vi "Hotel Room Service System.vi"() -> ()   [LabVIEW 2022 SP3]
uses:
  <vilib>/addons/control/pid/pid.llb/PID (DBL).vi
  <vilib>/addons/control/pid/NI_PID_pid.lvlib
panel:
  out "Emergency R2":bool
  in  "Smoke sensor":dbl(knob) scale=1.0..100.0 scale format="%#.6g"
  in  "Smoke sensor":dbl(knob) min=0.0 max=100.0 step=1.0 scale=0.0..100.0 scale format="%#.2g"
  in  "?":T1
  out "Password 3":string
  out "String 3":string
  out "Slide 2":u8(slide) scale=0.0..100.0
  in  "Search Button 2":bool
  out "Emergency R1":bool
  in  "Password 2":T1
  out "Password":string
  out "String 2":string
  out "Slide":u8(slide) scale=0.0..100.0
  in  "Search Button":bool
  in  "?":bool
  in  "Set point":dbl(slide)=15.0 min=15.0 max=30.0 step=1.0 scale=15.0..30.0
  in  "Room Tempreature":dbl(slide) scale=0.0..40.0
  out "System Action":string
  out "AC 3":bool
  out "Heator 6":bool
  in  "Set point":dbl(slide)=15.0 min=15.0 max=30.0 step=1.0 scale=15.0..30.0
  out "Heator":bool
  out "AC":bool
  out "System Action":string
  in  "A":dbl(slide) caption="Room Tempreature" min=0.0 max=45.0 step=1.0 scale=0.0..50.0
  in  "?":bool
  out "Your Order will be Prepared in":dbl
  out "R2":bool
  in  "Pay Bill and Conform":bool
  in  "Cheesecake":bool
  in  "Quantity":dbl=1.0 min=1.0 max=10.0 step=1.0
  out "Price":dbl
  in  "Chocolate Cake":bool
  in  "Quantity":dbl=1.0 min=1.0 max=10.0 step=1.0
  out "Price":dbl
  out "Total Bill":dbl
  out "Discount":string
  out "Order":string
  out "Order":string
  out "R1":bool
  out "Your Order will be Prepared in":dbl
  in  "Pay Bill and Conform":bool
  out "Discount":string
  out "Total Bill":dbl
  out "Price":dbl
  in  "Quantity 4":dbl=1.0 min=1.0 max=10.0 step=1.0
  in  "Chocolate Cake":bool
  out "Price":dbl
  in  "Quantity 3":dbl=1.0 min=1.0 max=10.0 step=1.0
  in  "Cheesecake":bool
  # "Hotel Room Service System"
  # "Customer Display"
  # "Hotel Display"
  # "Room 1"
  # "Foods"
  # "Room Tempreature Control"
  # "Room 2"
  # "Door Lock control"
  # "Door Lock control"
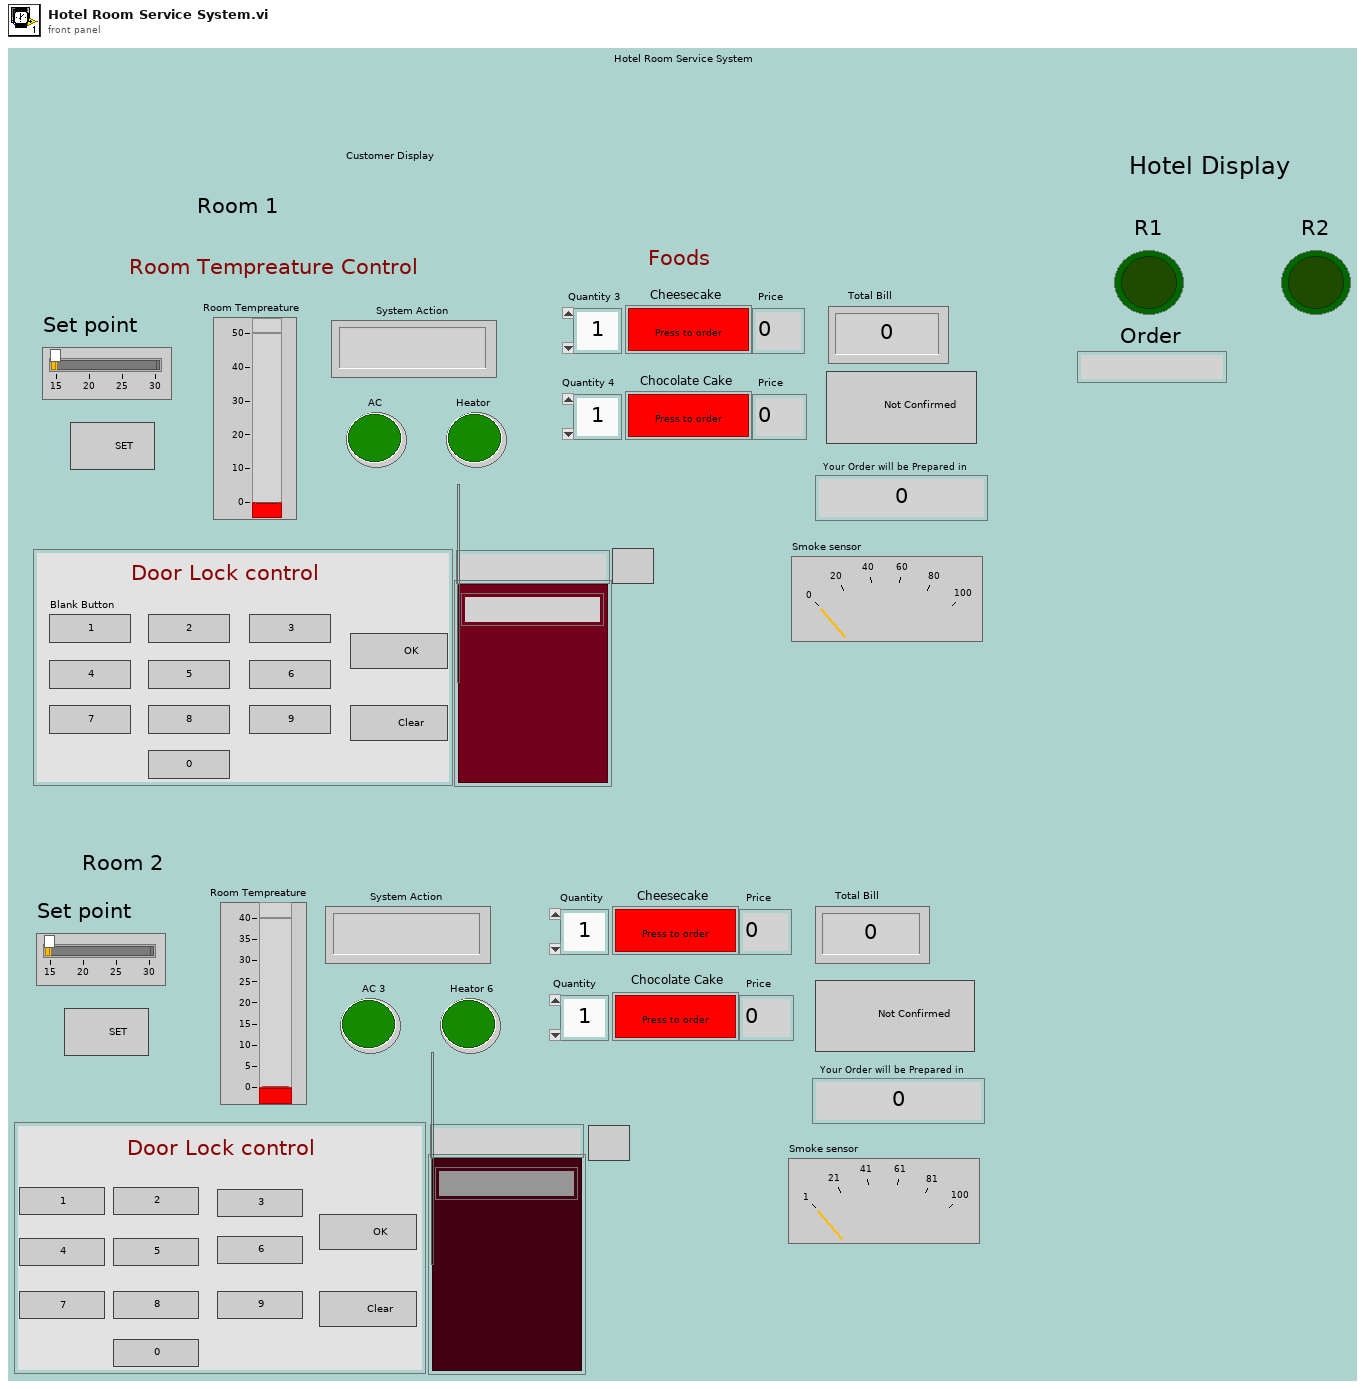
[diagram p1: front panel]
types:
  T1 = cluster{"Blank Button":bool, "Blank Button 2":bool, "Blank Button 3":bool, "Blank Button 4":bool, "Blank Button 5":bool, "Blank Button 6":bool, "Blank Button 7":bool, "Blank Button 8":bool, "Blank Button 9":bool, "Blank Button 10":bool, "OK Button":bool, "Refresh Button":bool}
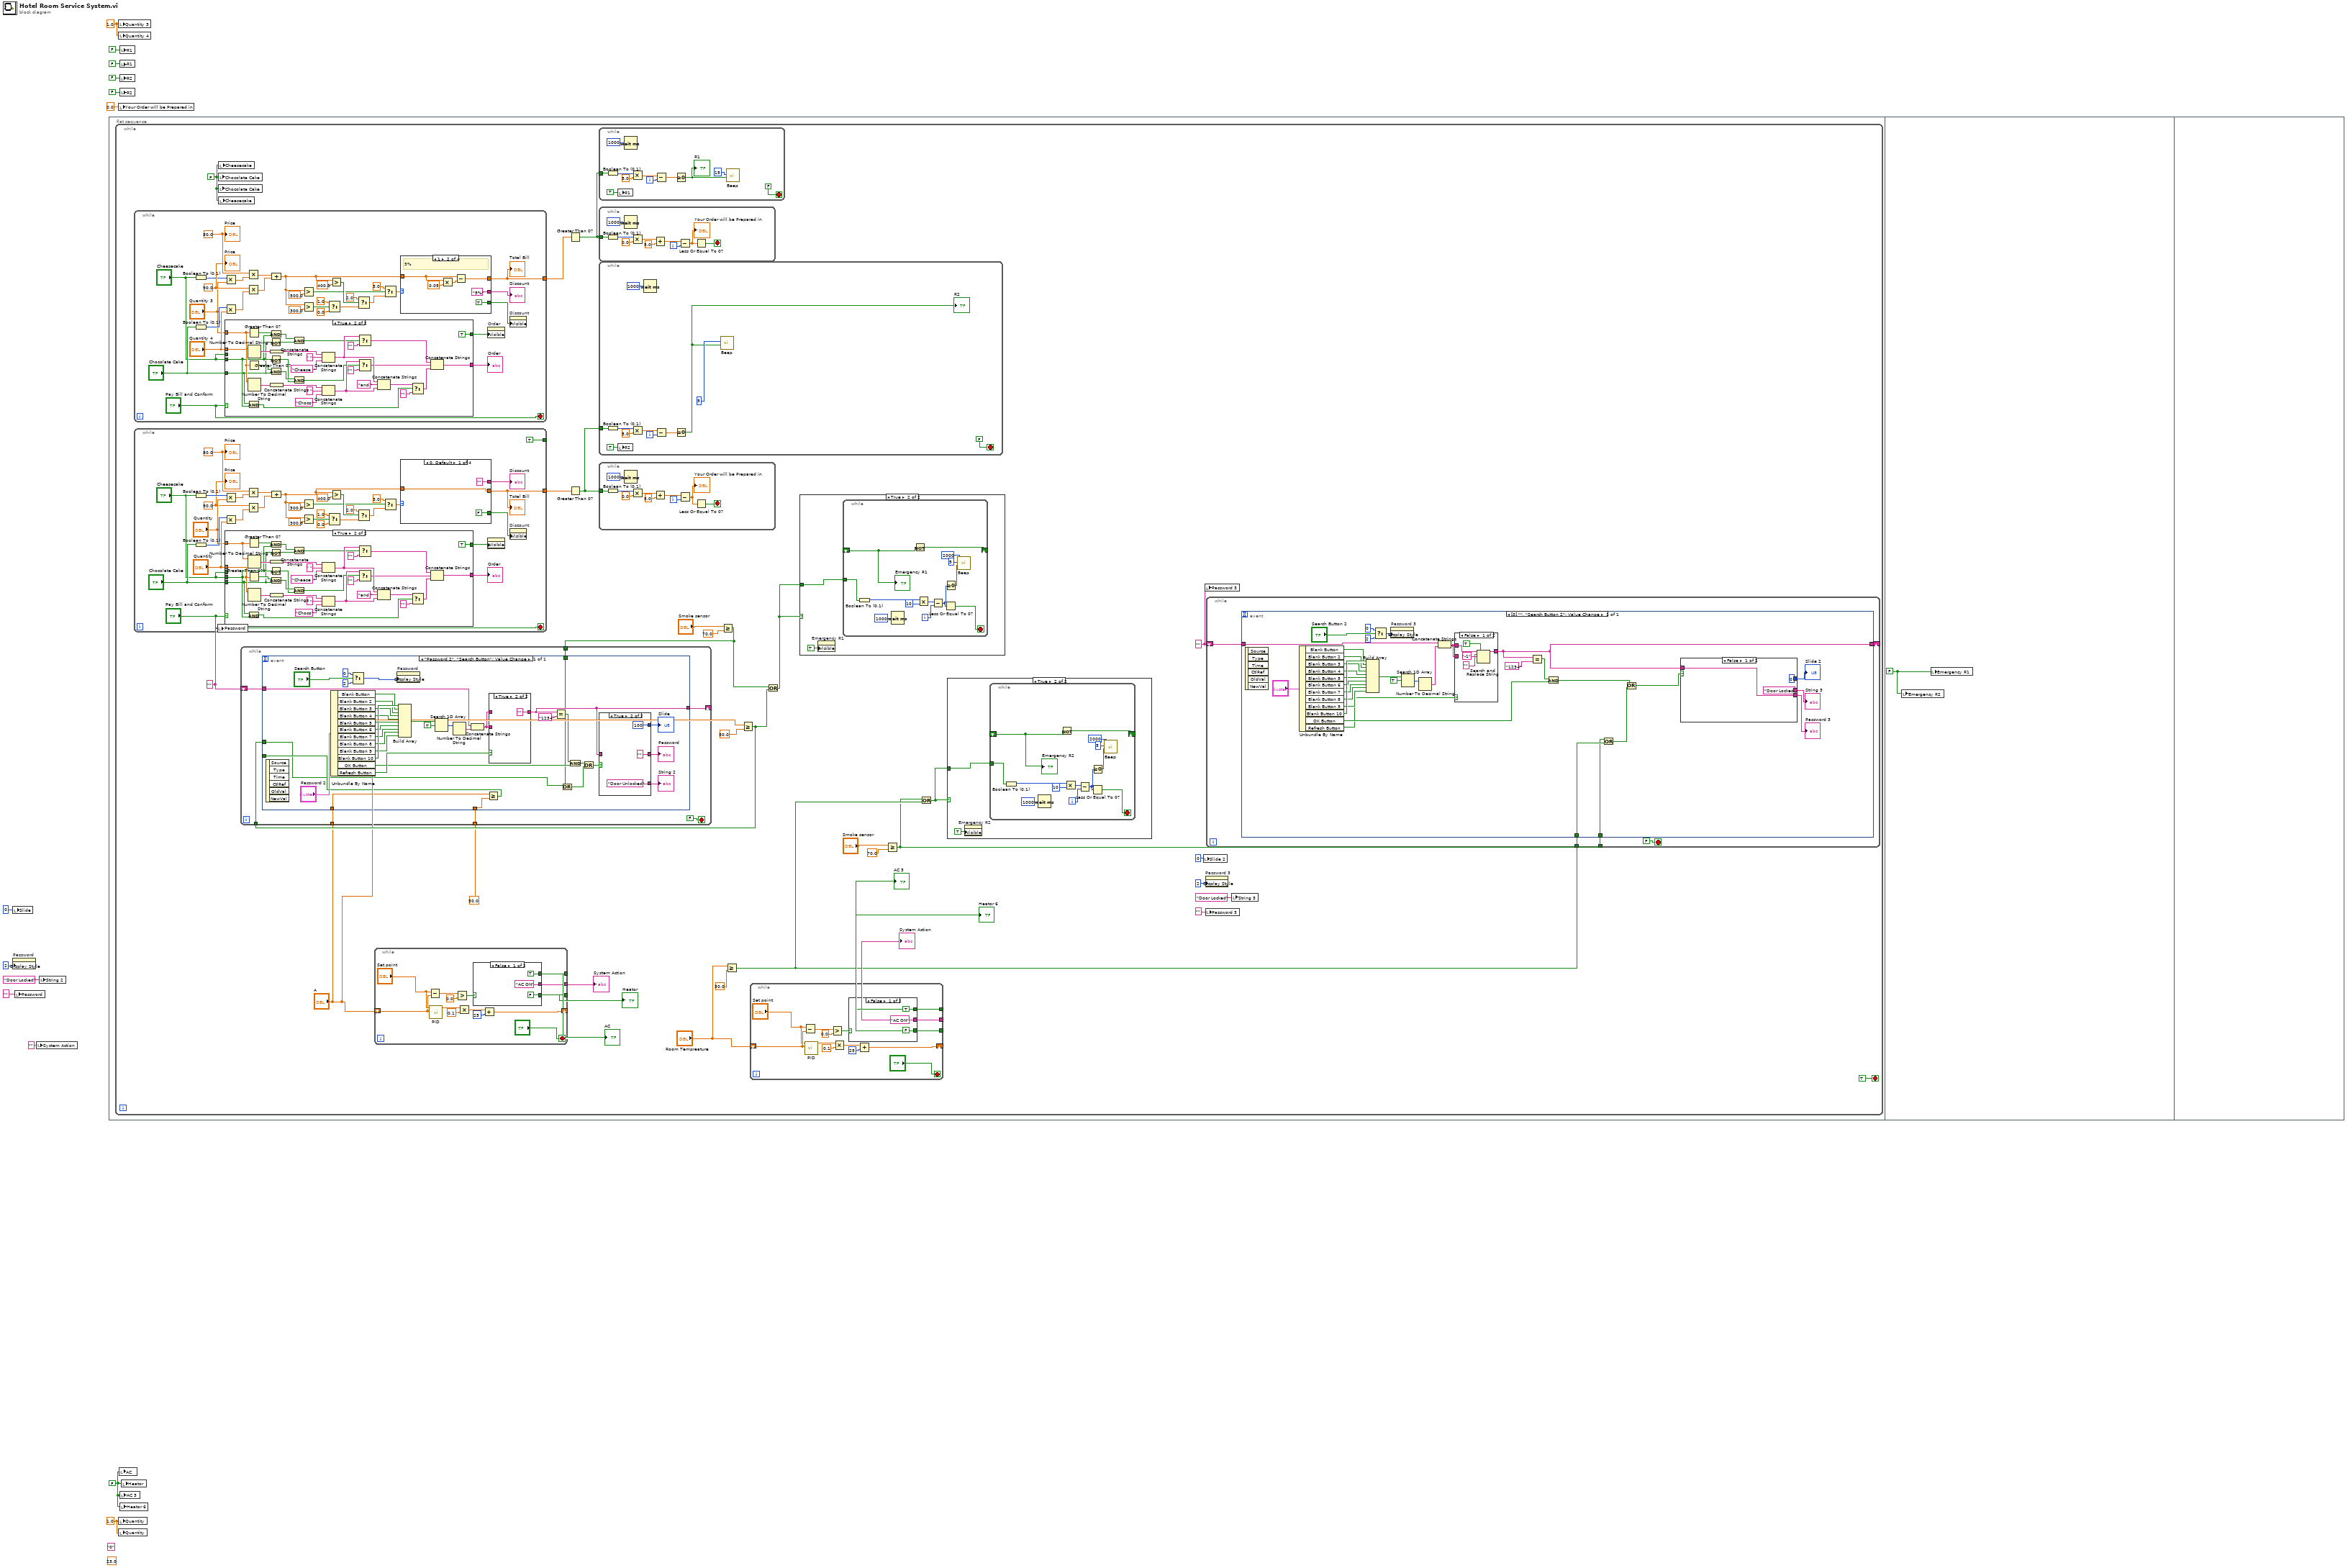
[diagram p0: block diagram]
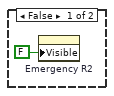
[diagram p2: hidden frame]
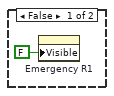
[diagram p3: hidden frame]
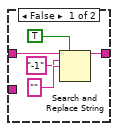
[diagram p4: hidden frame]
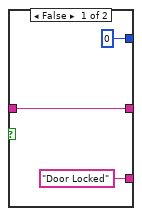
[diagram p5: hidden frame]
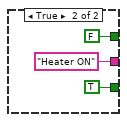
[diagram p6: hidden frame]
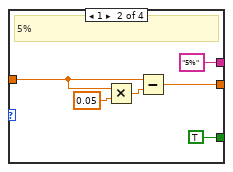
[diagram p7: hidden frame]
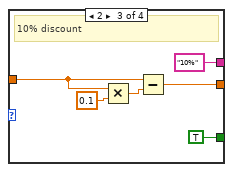
[diagram p8: hidden frame]
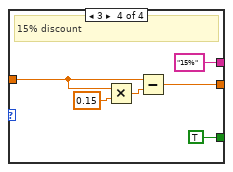
[diagram p9: hidden frame]
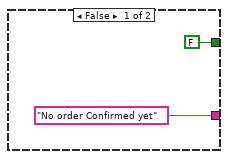
[diagram p10: hidden frame]
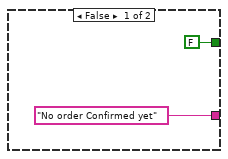
[diagram p11: hidden frame]
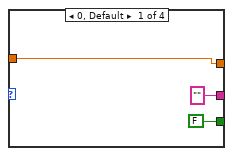
[diagram p12: hidden frame]
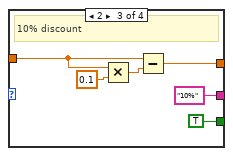
[diagram p13: hidden frame]
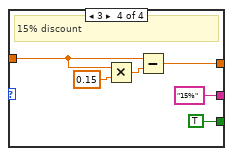
[diagram p14: hidden frame]
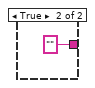
[diagram p15: hidden frame]
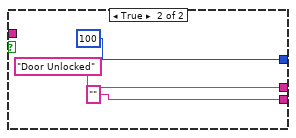
[diagram p16: hidden frame]
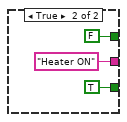
[diagram p17: hidden frame]
diagram:
  w6 = FALSE
  (unwired) 23.0 ("Target Temprature")
  (unwired) "0" ("Final")
  w9 = 1.0 ("Your Order will be Prepared in")
  w12 = 1.0 ("Your Order will be Prepared in")
  n1 = local write "Slide"(u8 0 ("Slide")) -> ()
  n2 = property on="Password" class="Str"("Display Style"=u32 2) -> ()  [unwired: 2 in, 2 out]
  n3 = local write "Password"("" ("Password")) -> ()
  n4 = local write "System Action"("" ("System Action")) -> ()
  n5 = local write "String 2"("Door Locked" ("String 2")) -> ()
  n6 = flat-sequence {
    frame #0 {
      n7 = while {
        stop <- TRUE stop-if-true
        w32 = ""
        w35 = ""
        w45 = FALSE ("Item 1")
        n8 = while {
          tunnel: [w295] -> w46
          stop <- "Pay Bill and Conform" stop-if-true
          w314 = 90.0 ("Price")
          w317 = 80.0 ("Price")
          n9 = Boolean To (0,1)(Boolean="Cheesecake") -> (0, 1=w294:i16)
          n10 = Boolean To (0,1)(Boolean="Chocolate Cake") -> (0, 1=w316:i16)
          n11 = Multiply(x=w294, y="Quantity 3") -> (x*y=w292:dbl)
          n12 = Multiply(x=w316, y="Quantity 4") -> (x*y=w315:dbl)
          n13 = case shown="True" "Pay Bill and Conform" {
            tunnel: ["No order Confirmed yet" w351] -> w293
            tunnel: "Quantity 4" -> [_ w347]
            tunnel: [FALSE TRUE ("Visible")] -> w291
            tunnel: "Quantity 3" -> [_ w329]
            tunnel: "Cheesecake" -> [_ _]
            tunnel: "Chocolate Cake" -> [_ w320]
            tunnel: "Cheesecake" -> [_ w321]
            frame False {
            }
            frame True {
              n14 = Greater Than 0?(x=w329) -> (x > 0?=w339:bool)
              n15 = Greater Than 0?(x=w347) -> (x > 0?=w338:bool)
              n16 = And(x=w320, y=w321) -> (x .and. y?=w337:bool)
              n17 = Number To Decimal String(number=w329) -> (decimal integer string=w350:string)  [unwired: 1 in]
              n18 = Number To Decimal String(number=w347) -> (decimal integer string=w349:string)  [unwired: 1 in]
              n19 = And(x=w339, y=w321) -> (x .and. y?=w325:bool)
              n20 = Not(x=w320) -> (.not. x?=w324:bool)
              n21 = Not(x=w321) -> (.not. x?=w328:bool)
              n22 = And(x=w338, y=w320) -> (x .and. y?=w330:bool)
              n23 = Concatenate Strings(w350) -> (w344:string)
              n24 = Concatenate Strings(w349) -> (w346:string)
              n25 = And(x=w325, y=w324) -> (x .and. y?=w323:bool)
              n26 = And(x=w330, y=w328) -> (x .and. y?=w322:bool)
              n27 = Concatenate Strings(w344, " ", "Cheese  ") -> (w335:string)
              n28 = Concatenate Strings(w346, " ", "Choco") -> (w333:string)
              n29 = Select(t=w335, s=w323, f="") -> (s? t:f=w327:string)
              n30 = Select(t=w333, s=w322, f="") -> (s? t:f=w326:string)
              n31 = Concatenate Strings(w335, "and ", w333) -> (w332:string)
              n32 = Select(t=w332, s=w337, f="") -> (s? t:f=w331:string)
              n33 = Concatenate Strings(w327, w326, w331) -> (w351:string)
            }
          }
          "Order" <- w293
          n34 = Multiply(x=w317, y=w292) -> (x*y=w313:dbl)
          n35 = Multiply(x=w314, y=w315) -> (x*y=w312:dbl)
          n36 = Compound Arithmetic op=ADD(w313, w312) -> (w298:dbl)
          n37 = Greater?(x=w298, y=500.0) -> (0:w300:bool)
          n38 = Greater?(x=w298, y=300.0) -> (0:w308:bool)
          n39 = Select(t=1.0, s=w308, f=0.0) -> (s? t:f=w303:dbl)
          n40 = Greater?(x=w298, y=400.0) -> (0:w305:bool)
          n41 = Select(t=2.0, s=w305, f=w303) -> (s? t:f=w301:dbl)
          n42 = Select(t=3.0, s=w300, f=w301) -> (s? t:f=w299:dbl)
          n43 = case shown="1" w299 {
            tunnel: w298 -> [w353 w359 w365 w371]
            tunnel: ["" ("Discount") "5%" ("Discount") "10%" ("Discount") "15%" ("Discount")] -> w297
            tunnel: [FALSE ("Visible") TRUE ("Visible") TRUE ("Visible") TRUE ("Visible")] -> w296
            tunnel: [w353 w356 w362 w368] -> w295
            frame 0, Default {
            }
            frame 1 {
              # "5%"
              n44 = Multiply(x=w359, y=0.05) -> (x*y=w360:dbl)
              n45 = Subtract(x=w359, y=w360) -> (x-y=w356:dbl)
            }
            frame 2 {
              # "10% discount"
              n46 = Multiply(x=w365, y=0.1) -> (x*y=w367:dbl)
              n47 = Subtract(x=w365, y=w367) -> (x-y=w362:dbl)
            }
            frame 3 {
              # "15% discount"
              n48 = Multiply(x=w371, y=0.15) -> (x*y=w373:dbl)
              n49 = Subtract(x=w371, y=w373) -> (x-y=w368:dbl)
            }
          }
          "Total Bill" <- w295
          "Discount" <- w297
          n50 = property on="Order" class="Str"("Visible"=w291) -> ()  [unwired: 2 in, 2 out]
          n51 = property on="Discount" class="Str"("Visible"=w296) -> ()  [unwired: 2 in, 2 out]
          "Price" <- w317
          "Price" <- w314
        }
        n52 = while {
          tunnel: [TRUE ("x")] -> _
          tunnel: [w197] -> w42
          stop <- "Pay Bill and Conform" stop-if-true
          w201 = 90.0 ("Price")
          w200 = 80.0 ("Price")
          n53 = Boolean To (0,1)(Boolean="Cheesecake") -> (0, 1=w216:i16)
          n54 = Boolean To (0,1)(Boolean="Chocolate Cake") -> (0, 1=w225:i16)
          n55 = Multiply(x=w216, y="Quantity") -> (x*y=w214:dbl)
          n56 = Multiply(x=w225, y="Quantity") -> (x*y=w224:dbl)
          n57 = case shown="True" "Pay Bill and Conform" {
            tunnel: ["No order Confirmed yet" w284] -> w215
            tunnel: "Quantity" -> [_ w280]
            tunnel: [FALSE TRUE ("Visible")] -> w213
            tunnel: "Quantity" -> [_ w262]
            tunnel: "Cheesecake" -> [_ _]
            tunnel: "Chocolate Cake" -> [_ w253]
            tunnel: "Cheesecake" -> [_ w254]
            frame False {
            }
            frame True {
              n58 = Greater Than 0?(x=w262) -> (x > 0?=w272:bool)
              n59 = Greater Than 0?(x=w280) -> (x > 0?=w271:bool)
              n60 = And(x=w253, y=w254) -> (x .and. y?=w270:bool)
              n61 = Number To Decimal String(number=w262) -> (decimal integer string=w283:string)  [unwired: 1 in]
              n62 = Number To Decimal String(number=w280) -> (decimal integer string=w282:string)  [unwired: 1 in]
              n63 = And(x=w272, y=w254) -> (x .and. y?=w258:bool)
              n64 = Not(x=w253) -> (.not. x?=w257:bool)
              n65 = Not(x=w254) -> (.not. x?=w261:bool)
              n66 = And(x=w271, y=w253) -> (x .and. y?=w263:bool)
              n67 = Concatenate Strings(w283) -> (w277:string)
              n68 = Concatenate Strings(w282) -> (w279:string)
              n69 = And(x=w258, y=w257) -> (x .and. y?=w256:bool)
              n70 = And(x=w263, y=w261) -> (x .and. y?=w255:bool)
              n71 = Concatenate Strings(w277, " ", "Cheese  ") -> (w268:string)
              n72 = Concatenate Strings(w279, " ", "Choco") -> (w266:string)
              n73 = Select(t=w268, s=w256, f="") -> (s? t:f=w260:string)
              n74 = Select(t=w266, s=w255, f="") -> (s? t:f=w259:string)
              n75 = Concatenate Strings(w268, "and ", w266) -> (w265:string)
              n76 = Select(t=w265, s=w270, f="") -> (s? t:f=w264:string)
              n77 = Concatenate Strings(w260, w259, w264) -> (w284:string)
            }
          }
          "Order" <- w215
          n78 = Multiply(x=w200, y=w214) -> (x*y=w223:dbl)
          n79 = Multiply(x=w201, y=w224) -> (x*y=w222:dbl)
          n80 = Compound Arithmetic op=ADD(w223, w222) -> (w226:dbl)
          n81 = Greater?(x=w226, y=500.0) -> (0:w217:bool)
          n82 = Greater?(x=w226, y=300.0) -> (0:w221:bool)
          n83 = Select(t=1.0, s=w221, f=0.0) -> (s? t:f=w219:dbl)
          n84 = Greater?(x=w226, y=400.0) -> (0:w220:bool)
          n85 = Select(t=2.0, s=w220, f=w219) -> (s? t:f=w218:dbl)
          n86 = Select(t=3.0, s=w217, f=w218) -> (s? t:f=w229:dbl)
          n87 = case shown="0, Default" w229 {
            tunnel: w226 -> [w230 w236 w242 w248]
            tunnel: ["" ("Discount") "5%" ("Discount") "10%" ("Discount") "15%" ("Discount")] -> w227
            tunnel: [FALSE ("Visible") TRUE ("Visible") TRUE ("Visible") TRUE ("Visible")] -> w228
            tunnel: [w230 w233 w239 w245] -> w197
            frame 0, Default {
            }
            frame 1 {
              # "5%"
              n88 = Multiply(x=w236, y=0.05) -> (x*y=w237:dbl)
              n89 = Subtract(x=w236, y=w237) -> (x-y=w233:dbl)
            }
            frame 2 {
              # "10% discount"
              n90 = Multiply(x=w242, y=0.1) -> (x*y=w244:dbl)
              n91 = Subtract(x=w242, y=w244) -> (x-y=w239:dbl)
            }
            frame 3 {
              # "15% discount"
              n92 = Multiply(x=w248, y=0.15) -> (x*y=w250:dbl)
              n93 = Subtract(x=w248, y=w250) -> (x-y=w245:dbl)
            }
          }
          "Total Bill" <- w197
          "Discount" <- w227
          n94 = property on="Order" class="Str"("Visible"=w213) -> ()  [unwired: 2 in, 2 out]
          n95 = property on="Discount" class="Str"("Visible"=w228) -> ()  [unwired: 2 in, 2 out]
          "Price" <- w200
          "Price" <- w201
        }
        n96 = local write "Password"(w35) -> ()
        n97 = local write "Chocolate Cake"(w45) -> ()
        n98 = local write "Chocolate Cake"(w45) -> ()
        n99 = local write "Cheesecake"(w45) -> ()
        n100 = local write "Cheesecake"(w45) -> ()
        n101 = while {
          shift-right: [w140] -> _
          shift-left: "A" -> [w135]
          tunnel: [w141] -> w41
          tunnel: [w139] -> w40
          tunnel: [w138] -> w39
          stop <- "?" stop-if-true
          n102 = Subtract(x="Set point", y=w135) -> (x-y=w144:dbl)
          n103 = call-poly <vilib>:"PID.vi"("process variable"=w135, "setpoint"="Set point") -> ("output"=w147:dbl)  [unwired: 8 in, 1 out]
          n104 = Greater?(x=w144, y=0.0) -> (0:w142:bool)
          n105 = Multiply(x=w147, y=0.1) -> (x*y=w146:dbl)
          n106 = case shown="False" w142 {
            tunnel: ["AC ON" "Heater ON"] -> w141
            tunnel: [TRUE FALSE] -> w139
            tunnel: [FALSE TRUE] -> w138
            frame False {
            }
            frame True {
            }
          }
          n107 = Add(x=w146, y=25) -> (x+y=w140:dbl)
        }
        "System Action" <- w41
        "AC" <- w40
        "Heator" <- w39
        n108 = Greater Than 0?(x=w46) -> (x > 0?=w44:bool)
        n109 = Greater Than 0?(x=w42) -> (x > 0?=w43:bool)
        n110 = while {
          tunnel: w44 -> [w165]
          i -> [w174]
          stop <- FALSE stop-if-true
          n111 = Boolean To (0,1)(Boolean=w165) -> (0, 1=w168:i16)
          n112 = local write "R1"(TRUE ("Kitchen")) -> ()
          n113 = Wait (ms)(milliseconds to wait=u32 1000) -> ()  [unwired: 1 out]
          n114 = Multiply(x=w168, y=5.0) -> (x*y=w167:dbl)
          n115 = Subtract(x=w167, y=w174) -> (x-y=w166:dbl)
          n116 = Greater Or Equal To 0?(x=w166) -> (x >= 0?=w171:bool)
          "R1" <- w171
          n117 = call <vilib>:"Beep.vi"("use system alert? (T)"=w171, "duration (msec)"=u32 15 ("milliseconds to wait")) -> ()  [unwired: 10 in]
        }
        n118 = while {
          tunnel: w44 -> [w155]
          i -> [w164]
          stop <- w160 stop-if-true
          n119 = Boolean To (0,1)(Boolean=w155) -> (0, 1=w156:i16)
          n120 = Wait (ms)(milliseconds to wait=u32 1000) -> ()  [unwired: 1 out]
          n121 = Multiply(x=w156, y=0.0) -> (x*y=w158:dbl)
          n122 = Add(x=w158, y=5.0) -> (x+y=w159:dbl)
          n123 = Subtract(x=w159, y=w164) -> (x-y=w157:dbl)
          "Your Order will be Prepared in" <- w157
          n124 = Less Or Equal To 0?(x=w157) -> (x <= 0?=w160:bool)
        }
        n125 = while {
          tunnel: w43 -> [w191]
          i -> [w194]
          stop <- FALSE stop-if-true
          n126 = Boolean To (0,1)(Boolean=w191) -> (0, 1=w192:i16)
          n127 = local write "R2"(TRUE) -> ()
          n128 = Multiply(x=w192, y=5.0) -> (x*y=w190:dbl)
          n129 = Wait (ms)(milliseconds to wait=u32 1000) -> ()  [unwired: 1 out]
          n130 = Subtract(x=w190, y=w194) -> (x-y=w188:dbl)
          n131 = Greater Or Equal To 0?(x=w188) -> (x >= 0?=w187:bool)
          "R2" <- w187
          n132 = call <vilib>:"Beep.vi"("use system alert? (T)"=w187, "duration (msec)"=u32 5 ("milliseconds to wait")) -> ()  [unwired: 10 in]
        }
        n133 = while {
          tunnel: w43 -> [w177]
          i -> [w185]
          stop <- w182 stop-if-true
          n134 = Boolean To (0,1)(Boolean=w177) -> (0, 1=w176:i16)
          n135 = Wait (ms)(milliseconds to wait=u32 1000) -> ()  [unwired: 1 out]
          n136 = Multiply(x=w176, y=0.0) -> (x*y=w180:dbl)
          n137 = Add(x=w180, y=5.0) -> (x+y=w181:dbl)
          n138 = Subtract(x=w181, y=w185) -> (x-y=w179:dbl)
          "Your Order will be Prepared in" <- w179
          n139 = Less Or Equal To 0?(x=w179) -> (x <= 0?=w182:bool)
        }
        n140 = Greater Or Equal?(x="Smoke sensor", y=70.0) -> (x >= y?=w21:bool)
        n141 = Greater Or Equal?(x="Room Tempreature", y=50.0 ("x")) -> (x >= y?=w17:bool)
        n142 = Greater Or Equal?(x="A", y=50.0) -> (x >= y?=w33:bool)
        n143 = while {
          shift-right: [w83] -> _
          shift-left: w35 -> [w84]
          tunnel: w33 -> [w82]
          tunnel: 50.0 ("y") -> [w81]
          tunnel: "A" -> [w80]
          tunnel: w21 -> [w79]
          stop <- FALSE stop-if-true
          n144 = event shown="[0] \"Password 2\", \"Search Button\": Value Change" {
            selector: _ -> [_]
            dyn-events: _ -> [_]
            timeout: _ -> [_]
            tunnel: w84 -> [w107]
            tunnel: [w100] -> w83
            tunnel: [w89] -> _
            tunnel: w82 -> [w88]
            tunnel: w81 -> [w91]
            tunnel: w80 -> [w90]
            tunnel: w79 -> [w87]
            event "Password 2", "Search Button": Value Change {
              n145 = event-data() -> ()  [unwired: 1 in, 6 out]
              n146 = Unbundle By Name("Password 2") -> ("Blank Button"=w120:bool, "Blank Button 2"=w119:bool, "Blank Button 3"=w118:bool, "Blank Button 4"=w117:bool, "Blank Button 5"=w116:bool, "Blank Button 6"=w115:bool, "Blank Button 7"=w114:bool, "Blank Button 8"=w113:bool, "Blank Button 9"=w112:bool, "Blank Button 10"=w121:bool, "OK Button"=w93:bool, "Refresh Button"=w102:bool)
              n147 = Select(t=u8 0 ("Slide"), s="Search Button", f=u8 2 ("Slide")) -> (s? t:f=w96:u8)
              n148 = property on="Password" class="Str"("Display Style"=w96) -> ()  [unwired: 2 in, 2 out]
              n149 = Build Array(w121, w120, w119, w118, w117, w116, w115, w114, w113, w112) -> (w111:bool[])
              n150 = Search 1D Array(1D array=w111, element=TRUE) -> (index of element=w109:i32)  [unwired: 1 in]
              n151 = Number To Decimal String(number=w109) -> (decimal integer string=w108:string)  [unwired: 1 in]
              n152 = Concatenate Strings(w107, w108) -> (w103:string)
              n153 = Greater Or Equal?(x=w90, y=w91) -> (x >= y?=w89:bool)
              n154 = case shown="True" w102 {
                tunnel: w103 -> [_ _]
                tunnel: w103 -> [w124 _]
                tunnel: [w123 "" ("result string")] -> w100
                frame False {
                  n155 = Search and Replace String(replace all?=TRUE ("replace all? (F)"), input string=w124, search string="-1", replace string="" ("replace string (\"\")")) -> (result string=w123:string)  [unwired: 4 in, 3 out]
                }
                frame True {
                }
              }
              n156 = Equal?(x=w100, y="1234") -> (x = y?=w94:bool)
              n157 = Or(x=w88, y=w87) -> (x .or. y?=w86:bool)
              n158 = And(x=w94, y=w93) -> (x .and. y?=w92:bool)
              n159 = Or(x=w92, y=w86) -> (x .or. y?=w95:bool)
              n160 = case shown="True" w95 {
                tunnel: [u8 0 ("Slide") u8 100 ("Slide")] -> w105
                tunnel: ["Door Locked" ("String 2") "Door Unlocked" ("String 2")] -> w104
                tunnel: [w129 "" ("Password")] -> w101
                tunnel: w100 -> [w129 _]
                frame False {
                }
                frame True {
                }
              }
              "Password" <- w101
              "String 2" <- w104
              "Slide" <- w105
            }
          }
        }
        n161 = while {
          shift-right: [w429] -> _
          shift-left: "Room Tempreature" -> [w434]
          tunnel: [w430] -> w36
          tunnel: [w428] -> w37
          tunnel: [w427] -> w38
          stop <- "?" stop-if-true
          n162 = Subtract(x="Set point", y=w434) -> (x-y=w433:dbl)
          n163 = call-poly <vilib>:"PID.vi"("process variable"=w434, "setpoint"="Set point") -> ("output"=w437:dbl)  [unwired: 8 in, 1 out]
          n164 = Greater?(x=w433, y=0.0) -> (0:w431:bool)
          n165 = Multiply(x=w437, y=0.1) -> (x*y=w436:dbl)
          n166 = case shown="False" w431 {
            tunnel: ["AC ON" "Heater ON"] -> w430
            tunnel: [TRUE FALSE] -> w428
            tunnel: [FALSE TRUE] -> w427
            frame False {
            }
            frame True {
            }
          }
          n167 = Add(x=w436, y=25) -> (x+y=w429:dbl)
        }
        "System Action" <- w36
        "AC 3" <- w37
        "Heator 6" <- w38
        n168 = Or(x=w21, y=w33) -> (x .or. y?=w20:bool)
        n169 = case shown="True" w20 {
          tunnel: w20 -> [_ w64]
          frame False {
            n170 = property on="Emergency R1" class="Bool (strict)"("Visible"=FALSE) -> ()  [unwired: 2 in, 2 out]
          }
          frame True {
            n171 = property on="Emergency R1" class="Bool (strict)"("Visible"=TRUE) -> ()  [unwired: 2 in, 2 out]
            n172 = while {
              shift-right: [w78] -> _
              shift-left: _ -> [w77]
              tunnel: w64 -> [w66]
              i -> [w72]
              stop <- w71 stop-if-true
              n173 = Boolean To (0,1)(Boolean=w66) -> (0, 1=w75:i16)
              n174 = Wait (ms)(milliseconds to wait=u32 1000) -> ()  [unwired: 1 out]
              n175 = Not(x=w77) -> (.not. x?=w78:bool)
              n176 = Multiply(x=w75, y=i16 10) -> (x*y=w73:i16)
              n177 = Subtract(x=w73, y=w72) -> (x-y=w70:i32)
              n178 = Less Or Equal To 0?(x=w70) -> (x <= 0?=w71:bool)
              n179 = Greater Or Equal To 0?(x=w70) -> (x >= 0?=w69:bool)
              n180 = call <vilib>:"Beep.vi"("use system alert? (T)"=w69, "duration (msec)"=u32 5, "frequency (Hz)"=u32 2000) -> ()  [unwired: 9 in]
              "Emergency R1" <- w77
            }
          }
        }
        n181 = Greater Or Equal?(x="Smoke sensor", y=70.0) -> (x >= y?=w16:bool)
        n182 = Or(x=w16, y=w17) -> (x .or. y?=w15:bool)
        n183 = case shown="True" w15 {
          tunnel: w15 -> [_ w48]
          frame False {
            n184 = property on="Emergency R2" class="Bool (strict)"("Visible"=FALSE) -> ()  [unwired: 2 in, 2 out]
          }
          frame True {
            n185 = property on="Emergency R2" class="Bool (strict)"("Visible"=TRUE) -> ()  [unwired: 2 in, 2 out]
            n186 = while {
              shift-right: [w62] -> _
              shift-left: _ -> [w61]
              tunnel: w48 -> [w50]
              i -> [w56]
              stop <- w55 stop-if-true
              n187 = Boolean To (0,1)(Boolean=w50) -> (0, 1=w59:i16)
              n188 = Wait (ms)(milliseconds to wait=u32 1000) -> ()  [unwired: 1 out]
              n189 = Not(x=w61) -> (.not. x?=w62:bool)
              n190 = Multiply(x=w59, y=i16 10) -> (x*y=w57:i16)
              n191 = Subtract(x=w57, y=w56) -> (x-y=w54:i32)
              n192 = Less Or Equal To 0?(x=w54) -> (x <= 0?=w55:bool)
              n193 = Greater Or Equal To 0?(x=w54) -> (x >= 0?=w53:bool)
              n194 = call <vilib>:"Beep.vi"("use system alert? (T)"=w53, "duration (msec)"=u32 5, "frequency (Hz)"=u32 2000) -> ()  [unwired: 9 in]
              "Emergency R2" <- w61
            }
          }
        }
        n195 = local write "Slide 2"(u8 0 ("Slide")) -> ()
        n196 = local write "Password 3"(w32) -> ()
        n197 = property on="Password 3" class="Str"("Display Style"=u32 2) -> ()  [unwired: 2 in, 2 out]
        n198 = local write "Password 3"("" ("Password")) -> ()
        n199 = while {
          shift-right: [w377] -> _
          shift-left: w32 -> [w378]
          tunnel: w17 -> [w376]
          tunnel: w16 -> [w375]
          stop <- FALSE stop-if-true
          n200 = event shown="[0] \"\", \"Search Button 2\": Value Change" {
            selector: _ -> [_]
            dyn-events: _ -> [_]
            timeout: _ -> [_]
            tunnel: w378 -> [w397]
            tunnel: [w388] -> w377
            tunnel: w376 -> [w381]
            tunnel: w375 -> [w380]
            event "Search Button 2": Value Change {
              n201 = event-data() -> ()  [unwired: 1 in, 6 out]
              n202 = Unbundle By Name("?") -> ("Blank Button"=w410:bool, "Blank Button 2"=w409:bool, "Blank Button 3"=w408:bool, "Blank Button 4"=w407:bool, "Blank Button 5"=w406:bool, "Blank Button 6"=w405:bool, "Blank Button 7"=w404:bool, "Blank Button 8"=w403:bool, "Blank Button 9"=w402:bool, "Blank Button 10"=w411:bool, "OK Button"=w393:bool, "Refresh Button"=w390:bool)
              n203 = Build Array(w411, w410, w409, w408, w407, w406, w405, w404, w403, w402) -> (w401:bool[])
              n204 = Select(t=u8 0 ("Slide"), s="Search Button 2", f=u8 2 ("Slide")) -> (s? t:f=w384:u8)
              n205 = property on="Password 3" class="Str"("Display Style"=w384) -> ()  [unwired: 2 in, 2 out]
              n206 = Search 1D Array(1D array=w401, element=TRUE) -> (index of element=w399:i32)  [unwired: 1 in]
              n207 = Number To Decimal String(number=w399) -> (decimal integer string=w398:string)  [unwired: 1 in]
              n208 = Concatenate Strings(w397, w398) -> (w391:string)
              n209 = case shown="False" w390 {
                tunnel: w391 -> [_ _]
                tunnel: w391 -> [w414 _]
                tunnel: [w413 "" ("result string")] -> w388
                frame False {
                  n210 = Search and Replace String(replace all?=TRUE ("replace all? (F)"), input string=w414, search string="-1", replace string="" ("replace string (\"\")")) -> (result string=w413:string)  [unwired: 4 in, 3 out]
                }
                frame True {
                }
              }
              n211 = Equal?(x=w388, y="1234") -> (x = y?=w392:bool)
              n212 = And(x=w392, y=w393) -> (x .and. y?=w383:bool)
              n213 = Or(x=w380, y=w381) -> (x .or. y?=w379:bool)
              n214 = Or(x=w383, y=w379) -> (x .or. y?=w382:bool)
              n215 = case shown="False" w382 {
                tunnel: [u8 0 ("Slide") u8 100 ("Slide")] -> w395
                tunnel: ["Door Locked" ("String 2") "Door Unlocked" ("String 2")] -> w394
                tunnel: [w419 "" ("Password")] -> w389
                tunnel: w388 -> [w419 _]
                frame False {
                }
                frame True {
                }
              }
              "Password 3" <- w389
              "String 3" <- w394
              "Slide 2" <- w395
            }
          }
        }
        n216 = local write "String 3"("Door Locked" ("String 2")) -> ()
      }
    }
    frame #1 {
      w445 = FALSE ("Hotel Notify")
      n217 = local write "Emergency R2"(w445) -> ()
      n218 = local write "Emergency R1"(w445) -> ()
    }
    frame #2 {
    }
  }
  n219 = local write "Quantity 3"(w12) -> ()
  n220 = local write "Quantity 4"(w12) -> ()
  n221 = local write "Your Order will be Prepared in"(0.0 ("Your Order will be Prepared in")) -> ()
  n222 = local write "Quantity"(w9) -> ()
  n223 = local write "Quantity"(w9) -> ()
  n224 = local write "AC"(w6) -> ()
  n225 = local write "R1"(FALSE ("Visible")) -> ()
  n226 = local write "R1"(FALSE ("Kitchen")) -> ()
  n227 = local write "R2"(FALSE) -> ()
  n228 = local write "R2"(FALSE) -> ()
  n229 = local write "AC 3"(w6) -> ()
  n230 = local write "Heator 6"(w6) -> ()
  n231 = local write "Heator"(w6) -> ()
